vi "Load From File.vi"(8 "error in (no error)":errorcluster, 11 "Sudoku Class in":refnum<class "Sudoku Class.lvclass">) -> (0 "error out":errorcluster, 3 "Sudoku Class out":refnum<class "Sudoku Class.lvclass">)   [LabVIEW 2015, in "Sudoku Library.lvlib" / "Sudoku Class.lvclass"]
doc: "Created IvanLis by LabVIEW Portal\nProfile: http://labviewportal.org/memberlist.php?mode=viewprofile&u=987\neMail: IvanLisanov@gMail.com\nTelegram: https://t.me/IvanLis"
uses:
  Sudoku Class.lvclass
  Sudoku Class.lvclass/Sudoku Class.ctl
  Sudoku Library.lvlib
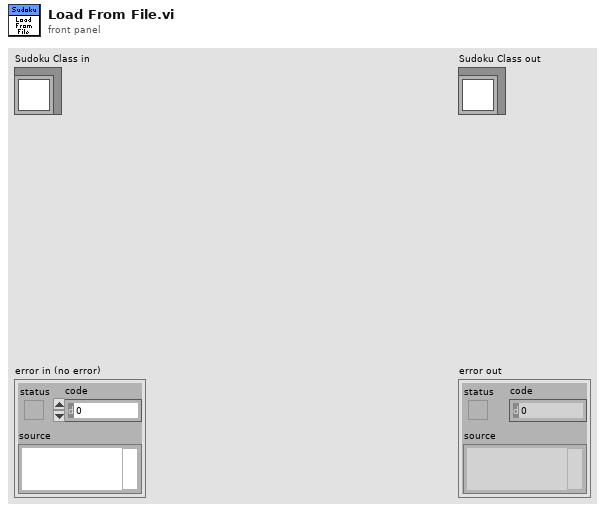
[diagram p1: front panel]
types:
  T1 = typedef "Sudoku Library.lvlib/Sudoku String.ctl" = string[][]
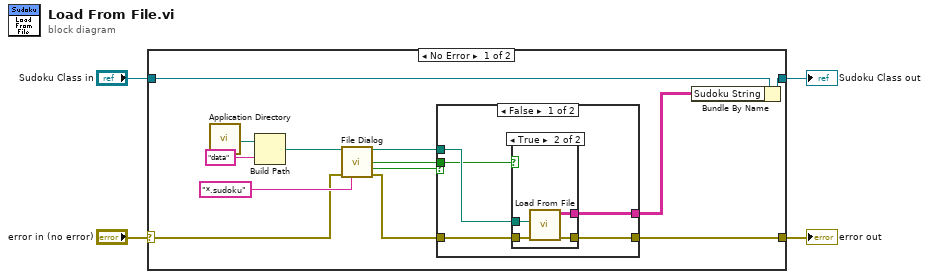
[diagram p0: block diagram]
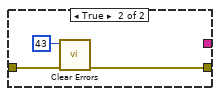
[diagram p3: hidden frame]
diagram:
  n1 = case shown="No Error" "error in (no error)" {
    selector: "error in (no error)" -> [w12 w32]
    tunnel: [w17 w32] -> w3
    tunnel: [w6 w31] -> w1
    tunnel: "Sudoku Class in" -> [w9 w31]
    frame No Error {
      n2 = call <vilib>:"Application Directory.vi"() -> ("Application Directory"=w15:path)
      n3 = Build Path(base path=w15, name or relative path="data") -> (appended path=w13:path)
      n4 = call "File Dialog"("start path"=w13, "error in"=w12, "pattern (all files)"="*.sudoku") -> ("selected path"=w8:path, "exists"=w7:bool, "cancelled"=w10:bool, "error out"=w11:errorcluster)  [unwired: 9 in]
      n5 = case shown="False" w10 {
        tunnel: [w22 w29] -> w17
        tunnel: w11 -> [w21 w30]
        tunnel: w8 -> [w20 _]
        tunnel: w7 -> [w19 _]
        tunnel: [w18 _] -> w5
        frame False {
          n6 = case shown="True" w19 {
            tunnel: [w23 w27] -> w22
            tunnel: w21 -> [w23 w26]
            tunnel: w20 -> [_ w25]
            tunnel: [_ w24] -> w18
            frame False {
            }
            frame True {
              n7 = call "Load From File.vi"("error in (no error)"=w26, "Sudoku File"=w25) -> ("error out"=w27:errorcluster, "Sudoku String"=w24:T1)  [unwired: 8 in]
            }
          }
        }
        frame True {
          n8 = call <vilib>:"Clear Errors.vi"("error in (no error)"=w30, "specific error code to clear (0: all)"=43) -> ("error out"=w29:errorcluster)  [unwired: 4 in, 1 out]
        }
      }
      n9 = Bundle By Name(cluster=w9, "Sudoku String"=w5) -> (w6:refnum<class "Sudoku Class.lvclass">)
    }
    frame Error {
    }
  }
  "error out" <- w3
  "Sudoku Class out" <- w1
